vi "SV Histogram from Element Data (1 Ch) (DBL).vi"(0 "new data":dbl, 1 "reset (F)":bool, 5 "range":cluster{"minimum":dbl, "maximum":dbl}={"minimum"=-10.0, "maximum"=10.0}, 7 "number of bins":i32=20) -> (4 "histogram":cluster{"bin centers":dbl[], "counts":u64[]}(graph), 6 "actual range":cluster{"minimum":dbl, "maximum":dbl}={"minimum"=-10.0, "maximum"=10.0}, 8 "counts":T1)   [LabVIEW 2017]
doc: "Use this VI to create a histogram of the input data. Set <B>range</B> and <B>number of bins</B> to specify the bins to include. Choose the appropriate instance based on the input data."
uses:
  <vilib>/addons/_NISVFA/_Shared subVIs/Controls/svc_Histogram Counts.ctl
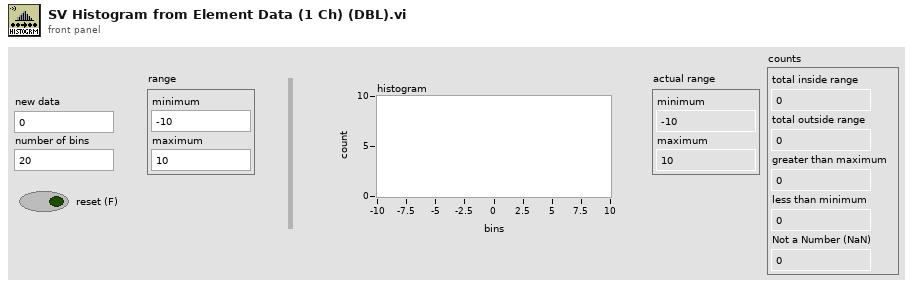
[diagram p1: front panel]
types:
  T1 = typedef "svc_Histogram Counts.ctl" = cluster{"total inside range":u64, "total outside range":u64, "greater than maximum":u64, "less than minimum":u64, "Not a Number (NaN)":u64}
  T2 = typedef "svc_Bin Specification.ctl" = cluster{"lower":dbl, "upper":dbl, "inclusion":u32}
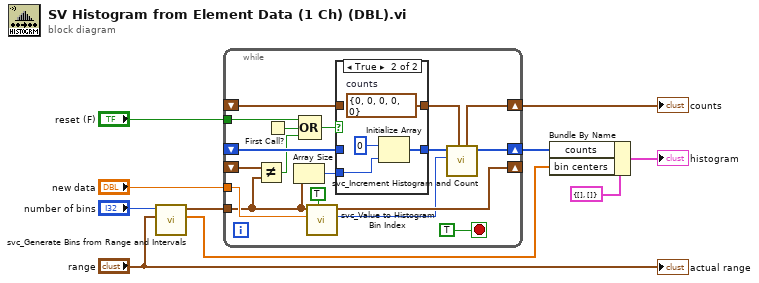
[diagram p0: block diagram]
diagram:
  n1 = call <vilib>:"svc_Generate Bins from Range and Intervals.vi"("range"="range", "number of bins"="number of bins") -> ("nominal centers"=w2:dbl[], "bins"=w8:T2[])  [unwired: 8 in]
  n2 = while {
    tunnel: "new data" -> [w20]
    tunnel: w8 -> [w18]
    shift-right: [w12] -> w4
    shift-left: _ -> [w26]
    shift-right: [w14] -> w1
    shift-left: _ -> [w27]
    shift-right: [w25] -> _
    shift-left: _ -> [w24]
    tunnel: "reset (F)" -> [w22]
    stop <- TRUE stop-if-true
    n3 = Not Equal?(x=w24, y=w18) -> (x != y?=w23:bool)
    n4 = First Call?() -> (First Call?: T/F=w17:bool)
    n5 = Array Size(array=w18) -> (size(s)=w19:i32)
    n6 = Compound Arithmetic op=OR(w22, w17, w23) -> (w21:bool)
    n7 = call <vilib>:"svc_Value to Histogram Bin Index.vi"("evenly spaced (F)"=TRUE, "value"=w20, "bins in"=w18) -> ("bin index"=w11:i32, "bins out"=w25:T2[])  [unwired: 7 in]
    n8 = case shown="True" w21 {
      tunnel: [w30 w34] -> w15
      tunnel: w27 -> [w30 _]
      tunnel: [w29 w32] -> w13
      tunnel: w26 -> [w29 _]
      tunnel: w19 -> [_ w31]
      frame False {
      }
      frame True {
        w34 = T1 {"total inside range"=0, "total outside range"=0, "greater than maximum"=0, "less than minimum"=0, "Not a Number (NaN)"=0}  # counts
        n9 = Initialize Array(u64 0 ("element"), w31) -> (w32:u64[])
      }
    }
    n10 = call <vilib>:"svc_Increment Histogram and Count.vi"("counts in"=w15, "bin index"=w11, "histogram in"=w13) -> ("histogram out"=w12:u64[], "counts out"=w14:T1)  [unwired: 7 in]
  }
  "counts" <- w1
  n11 = Bundle By Name(cluster=cluster{"bin centers":dbl[], "counts":u64[]} {"bin centers"=[], "counts"=[]}, "counts"=w4, "bin centers"=w2) -> (→"histogram":cluster{"bin centers":dbl[], "counts":u64[]})
  "actual range" <- "range"
